vi "故障提醒功能.vi"() -> (0 "以后不显示 2":bool)   [LabVIEW 2013]
panel:
  in  "退出":bool
  in  "以后不显示":bool
  in  "故码障解析":bool
  in  "结果":i32(listbox)=-1
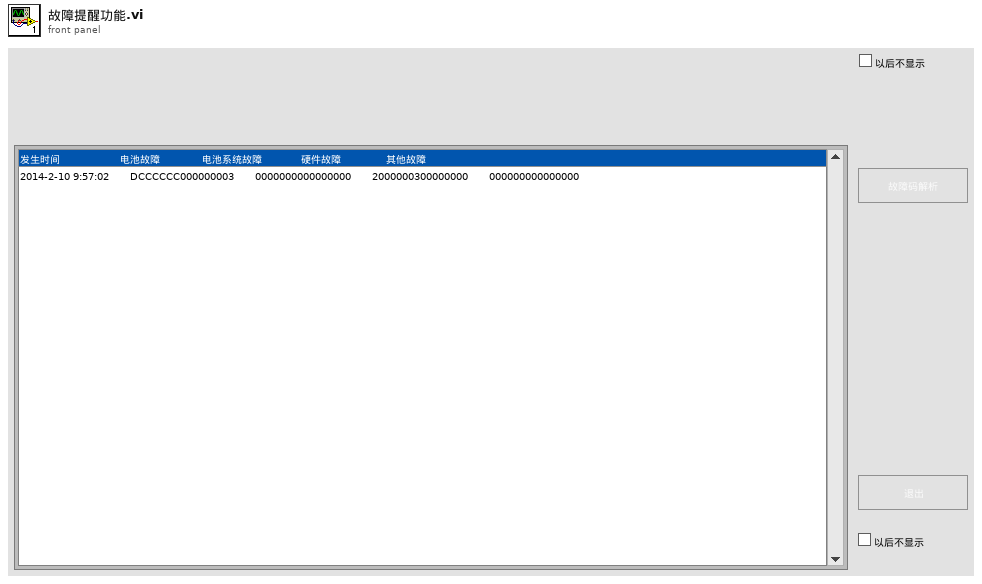
[diagram p1: front panel]
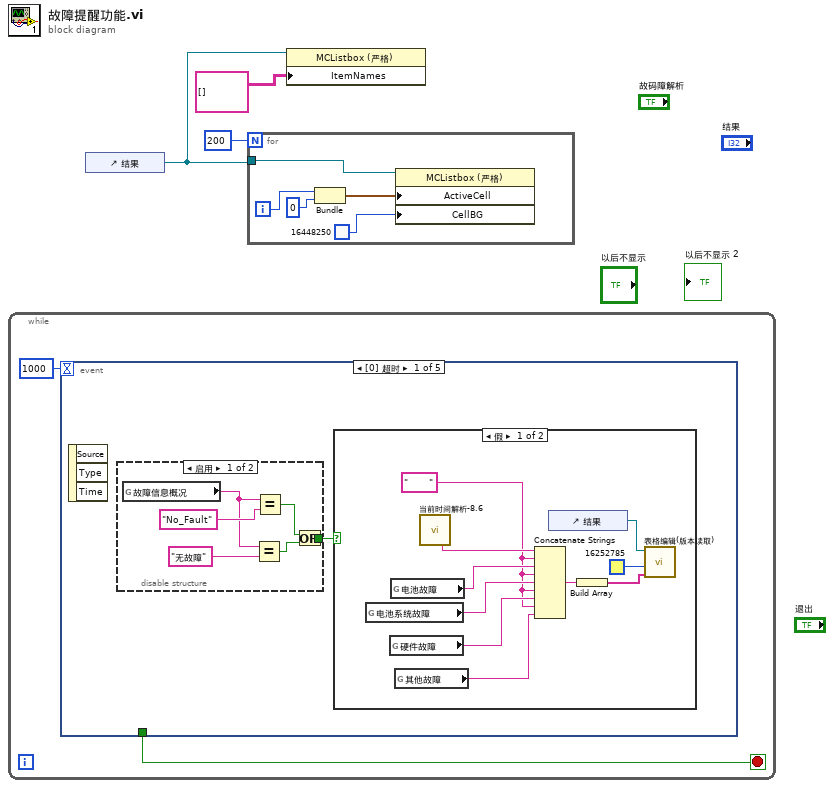
[diagram p0: block diagram]
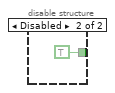
[diagram p2: hidden frame]
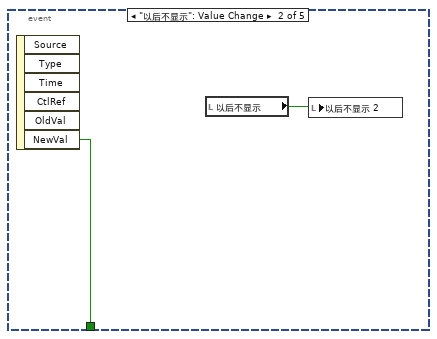
[diagram p4: hidden frame]
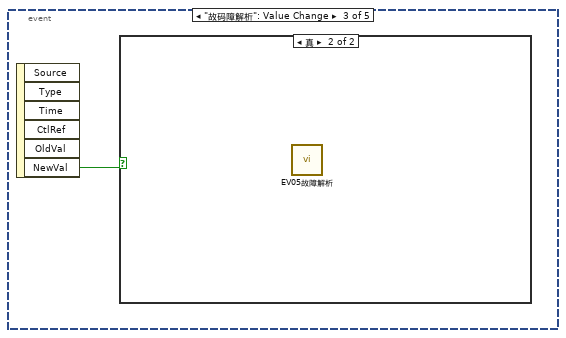
[diagram p5: hidden frame]
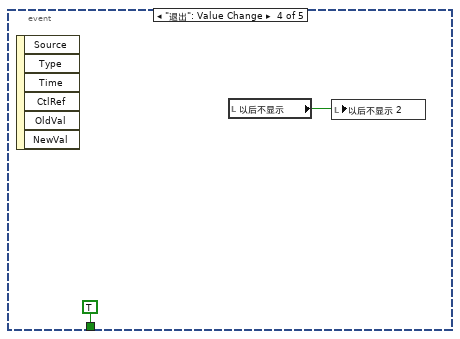
[diagram p7: hidden frame]
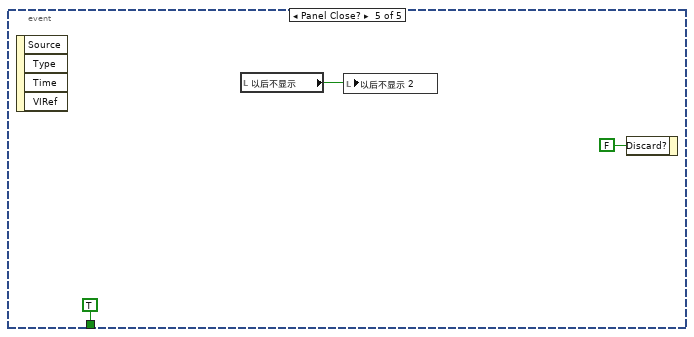
[diagram p8: hidden frame]
diagram:
  n1 = while {
    stop <- w4 stop-if-true
    n2 = event shown="[0] 超时" {
      selector: _ -> [_ _ _ _ _]
      dyn-events: _ -> [_ _ _ _ _]
      timeout: 1000 -> [_ _ _ _ _]
      tunnel: [_ w25 _ TRUE ("NewVal") TRUE ("NewVal")] -> w4
      event Timeout {
        n3 = event-data() -> ()  [unwired: 1 in, 3 out]
        n4 = disable-structure shown="启用" {
          disable-tunnel: [w7 TRUE] -> w6
          frame Enabled {
            n5 = global read "EV05全局变量1.vi" "故障信息概况"() -> (w8:string)
            n6 = Equal?(x=w8, y="无故障") -> (x = y?=w10:bool)
            n7 = Equal?(x=w8, y="No_Fault") -> (x = y?=w9:bool)
            n8 = Or(x=w9, y=w10) -> (x .or. y?=w7:bool)
          }
          frame Disabled {
          }
        }
        n9 = case shown="假" w6 {
          frame False {
            w17 = "       "
            n10 = global read "EV05全局变量1.vi" "电池系统故障"() -> (w20:string)
            n11 = global read "EV05全局变量1.vi" "硬件故障"() -> (w19:string)
            n12 = global read "EV05全局变量1.vi" "电池故障"() -> (w21:string)
            n13 = global read "EV05全局变量1.vi" "其他故障"() -> (w18:string)
            n14 = call "当前时间解析-8.6.vi"() -> ("时间"=w22:string)  [unwired: 10 in, 9 out]
            n15 = Concatenate Strings(w22, w17, w21, w17, w20, w17, w19, w17, w18) -> (w16:string)
            n16 = control-ref of="结果"() -> (w23:refnum<vi>)
            n17 = Build Array(w16) -> (w15:string[])
            n18 = call "表格编辑(版本读取).vi"("新元素/子数组"=w15, "活动单元格:单元格背景色"=u32 16252785, "MCListbox引用句柄"=w23) -> ()  [unwired: 1 in, 8 out]
          }
          frame True {
          }
        }
      }
      event "以后不显示": Value Change {
        n19 = event-data() -> ("NewVal"=w25:bool)  [unwired: 1 in, 5 out]
        n20 = local read "以后不显示"() -> (w24:bool)
        n21 = local write "以后不显示 2"(w24) -> ()
      }
      event "故码障解析": Value Change {
        n22 = event-data() -> ("NewVal"=w26:bool)  [unwired: 1 in, 5 out]
        n23 = case shown="真" w26 {
          frame False {
          }
          frame True {
            n24 = call "EV05故障解析.vi"() -> ()  [unwired: 12 in]
          }
        }
      }
      event "退出": Value Change {
        n25 = event-data() -> ()  [unwired: 1 in, 6 out]
        n26 = local read "以后不显示"() -> (w27:bool)
        n27 = local write "以后不显示 2"(w27) -> ()
      }
      event Panel Close? {
        n28 = event-data() -> ()  [unwired: 1 in, 4 out]
        n29 = local read "以后不显示"() -> (w29:bool)
        n30 = local write "以后不显示 2"(w29) -> ()
        n31 = event-data("Discard?"=FALSE ("放弃？")) -> ()  [unwired: 1 in, 1 out]
      }
    }
  }
  n32 = control-ref of="结果"() -> (w1:refnum<vi>)
  n33 = for {
    N: 200 -> [_]
    tunnel: w1 -> [w36]
    i -> [w34]
    n34 = Bundle(w34, 0) -> (w32:cluster{i32, i32})  [unwired: 1 out]
    n35 = property class="MCListbox (严格)"(reference=w36, "ActiveCell"=w32, "CellBG"=u32 16448250) -> ()  [unwired: 1 in, 2 out]
  }
  n36 = property class="MCListbox (严格)"(reference=w1, "ItemNames"=string[][] [] ("项名")) -> ()  [unwired: 1 in, 2 out]
